vi "NavX Motor Scalar.vi"(6 "Direction":enum16{"Left", "Right"}(ring), 10 "Yaw":dbl, 11 "Target Angle":dbl) -> (2 "Right Motor Out":dbl, 3 "Left Motor Out":dbl)   [LabVIEW 2015]
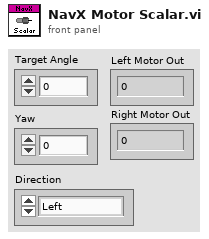
[diagram p1: front panel]
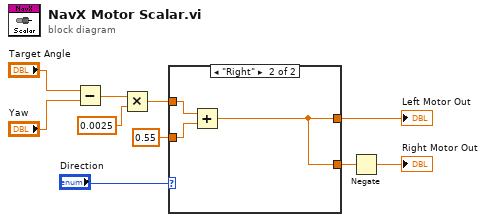
[diagram p0: block diagram]
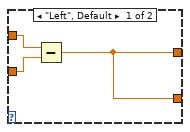
[diagram p2: hidden frame]
diagram:
  n1 = Subtract(x="Target Angle", y="Yaw") -> (x-y=w8:dbl)
  n2 = Multiply(x=w8, y=0.0025) -> (x*y=w6:dbl)
  n3 = case shown="\"Right\"" "Direction" {
    tunnel: w6 -> [w13 w16]
    tunnel: 0.55 -> [w12 w15]
    tunnel: [w11 w14] -> w3
    tunnel: [w11 w14] -> w2
    frame "Left", Default {
      n4 = Subtract(x=w13, y=w12) -> (x-y=w11:dbl)
    }
    frame "Right" {
      n5 = Add(x=w16, y=w15) -> (x+y=w14:dbl)
    }
  }
  "Left Motor Out" <- w3
  n6 = Negate(x=w2) -> (-x=→"Right Motor Out":dbl)
